vi "setClaseDB.vi"(8 "error in":errorcluster, 10 "claseDBValues":T1, 11 "claseDB in":refnum<class "claseDB.lvclass">) -> (0 "error out":errorcluster, 3 "claseDB out":refnum<class "claseDB.lvclass">)   [LabVIEW 2014, in "claseDB.lvclass"]
uses:
  claseDB.lvclass
  claseDB.lvclass/claseDB.ctl
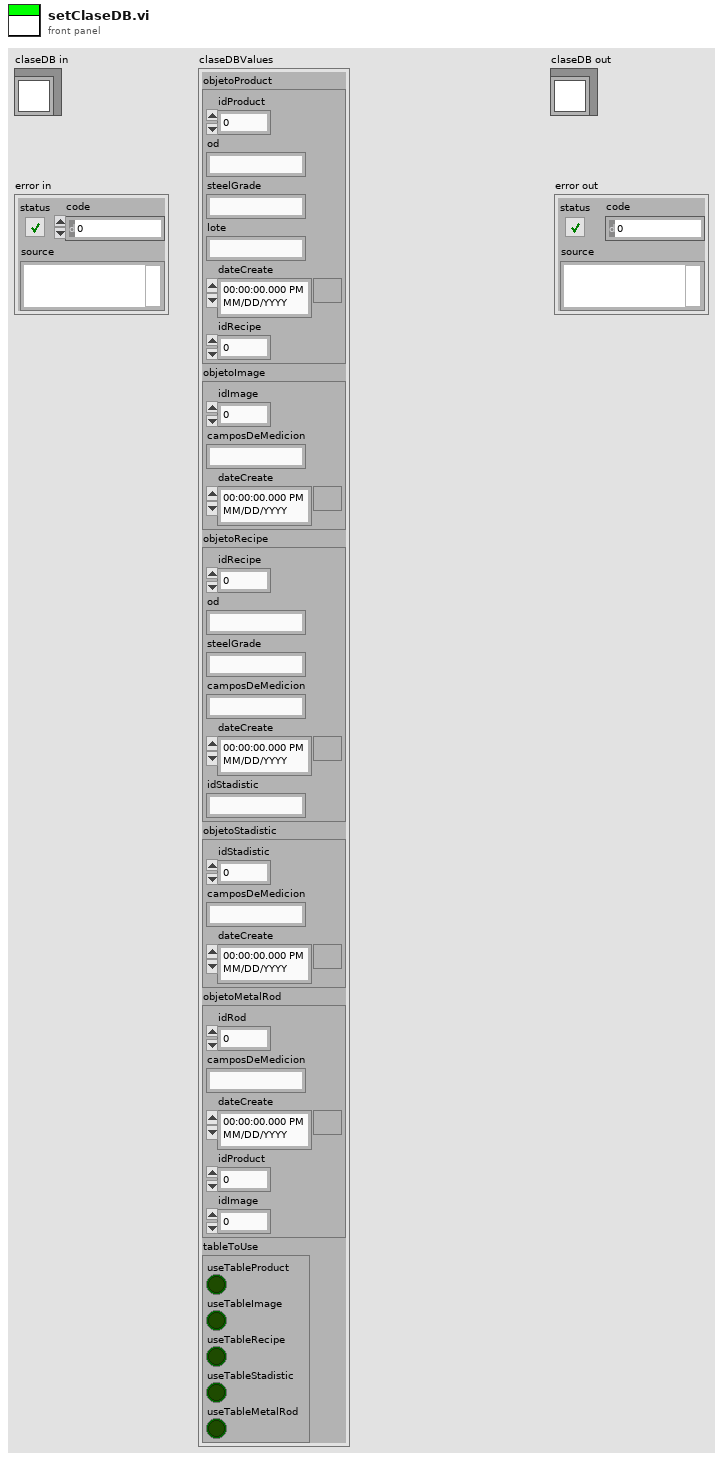
[diagram p1: front panel]
types:
  T1 = cluster{"objetoProduct":cluster{"idProduct":dbl, "od":string, "steelGrade":string, "lote":string, "dateCreate":timestamp, "idRecipe":dbl}, "objetoImage":cluster{"idImage":dbl, "camposDeMedicion":string, "dateCreate":timestamp}, "objetoRecipe":cluster{"idRecipe":dbl, "od":string, "steelGrade":string, "camposDeMedicion":string, "dateCreate":timestamp, "idStadistic":string}, "objetoStadistic":cluster{"idStadistic":dbl, "camposDeMedicion":string, "dateCreate":timestamp}, "objetoMetalRod":cluster{"idRod":dbl, "camposDeMedicion":string, "dateCreate":timestamp, "idProduct":dbl, "idImage":dbl}, "tableToUse":cluster{"useTableProduct":bool, "useTableImage":bool, "useTableRecipe":bool, "useTableStadistic":bool, "useTableMetalRod":bool}}
  T2 = cluster{"idProduct":dbl, "od":string, "steelGrade":string, "lote":string, "dateCreate":timestamp, "idRecipe":dbl}
  T3 = cluster{"idImage":dbl, "camposDeMedicion":string, "dateCreate":timestamp}
  T4 = cluster{"idRecipe":dbl, "od":string, "steelGrade":string, "camposDeMedicion":string, "dateCreate":timestamp, "idStadistic":string}
  T5 = cluster{"idStadistic":dbl, "camposDeMedicion":string, "dateCreate":timestamp}
  T6 = cluster{"idRod":dbl, "camposDeMedicion":string, "dateCreate":timestamp, "idProduct":dbl, "idImage":dbl}
  T7 = cluster{"useTableProduct":bool, "useTableImage":bool, "useTableRecipe":bool, "useTableStadistic":bool, "useTableMetalRod":bool}
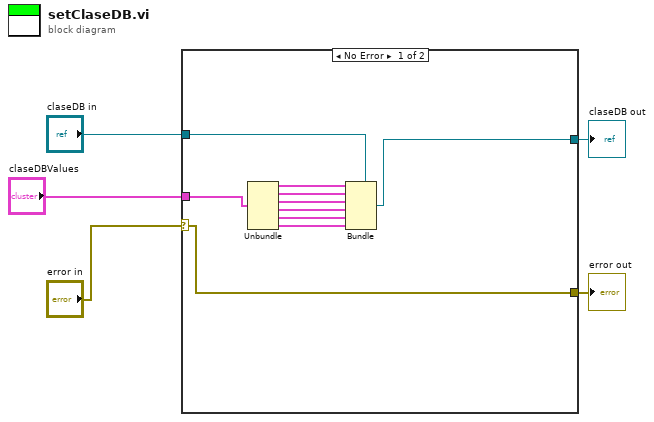
[diagram p0: block diagram]
diagram:
  n1 = case shown="No Error" "error in" {
    selector: "error in" -> [w14 w16]
    tunnel: "claseDB in" -> [w13 _]
    tunnel: [w15 _] -> w3
    tunnel: [w14 w16] -> w2
    tunnel: "claseDBValues" -> [w12 _]
    frame No Error {
      n2 = Unbundle(w12) -> ("objetoProduct"=w11:T2, "objetoImage"=w10:T3, "objetoRecipe"=w9:T4, "objetoStadistic"=w8:T5, "objetoMetalRod"=w7:T6, "tableToUse"=w6:T7)
      n3 = Bundle(cluster=w13, w11, w10, w9, w8, w7, w6) -> (w15:refnum<class "claseDB.lvclass">)
    }
    frame Error {
    }
  }
  "claseDB out" <- w3
  "error out" <- w2
